vi "get_system_paths.vi"(8 "error in (no error)":errorcluster) -> (0 "error out":errorcluster, 3 "paths []":path[](array[path]))   [LabVIEW 2015, in "lv-bin.lvlib" / "v1.lvlib"]
doc: "This vi can be used to get the system paths to add them to (add_data_path.vi) to maintain the use case for being able to use the absolute path or realtive path of your executable."
uses:
  v1.lvlib
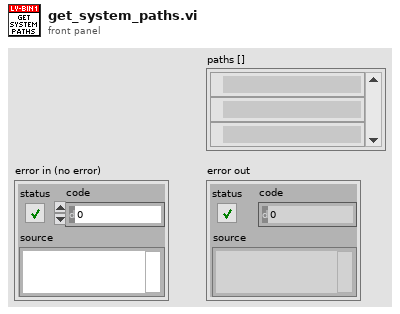
[diagram p1: front panel]
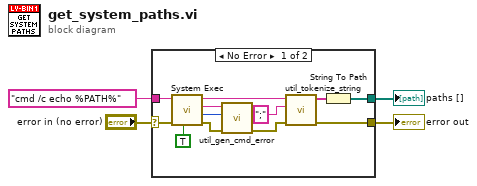
[diagram p0: block diagram]
diagram:
  n1 = case shown="No Error" "error in (no error)" {
    selector: "error in (no error)" -> [w10 w17]
    tunnel: [w9 w17] -> w3
    tunnel: [w5 _] -> w2
    tunnel: "cmd /c echo %PATH%" ("command line") -> [w7 _]
    frame No Error {
      n2 = call <vilib>:"System Exec.vi"("run minimized? (F)"=TRUE, "error in (no error)"=w10, "command line"=w7) -> ("error out"=w13:errorcluster, "return code"=w14:i32, "standard error"=w15:string, "standard output"=w16:string)  [unwired: 5 in]
      n3 = call "util_gen_cmd_error.vi"("error in (no error)"=w13, "return_code"=w14, "standard_error"=w15) -> ("error out"=w12:errorcluster)  [unwired: 8 in]
      n4 = call "util_tokenize_string.vi"("error in (no error)"=w12, "delimiter"=";", "input_string"=w16) -> ("error out"=w9:errorcluster, "before_match []"=w6:string[])  [unwired: 6 in, 1 out]
      n5 = String To Path(string=w6) -> (path=w5:path[])
    }
    frame Error {
    }
  }
  "error out" <- w3
  "paths []" <- w2
